vi "HEWH Data Cleanup at Index Location.vi"(10 "Test Data-Start to End IN":string[][](array[string]), 11 "Full Data DBL In":dbl[][](array[numeric])) -> (2 "Test Data-Start to End Out":string[][](array[string]), 3 "Full Data DBL Out":dbl[][](array[numeric]))   [LabVIEW 2020]
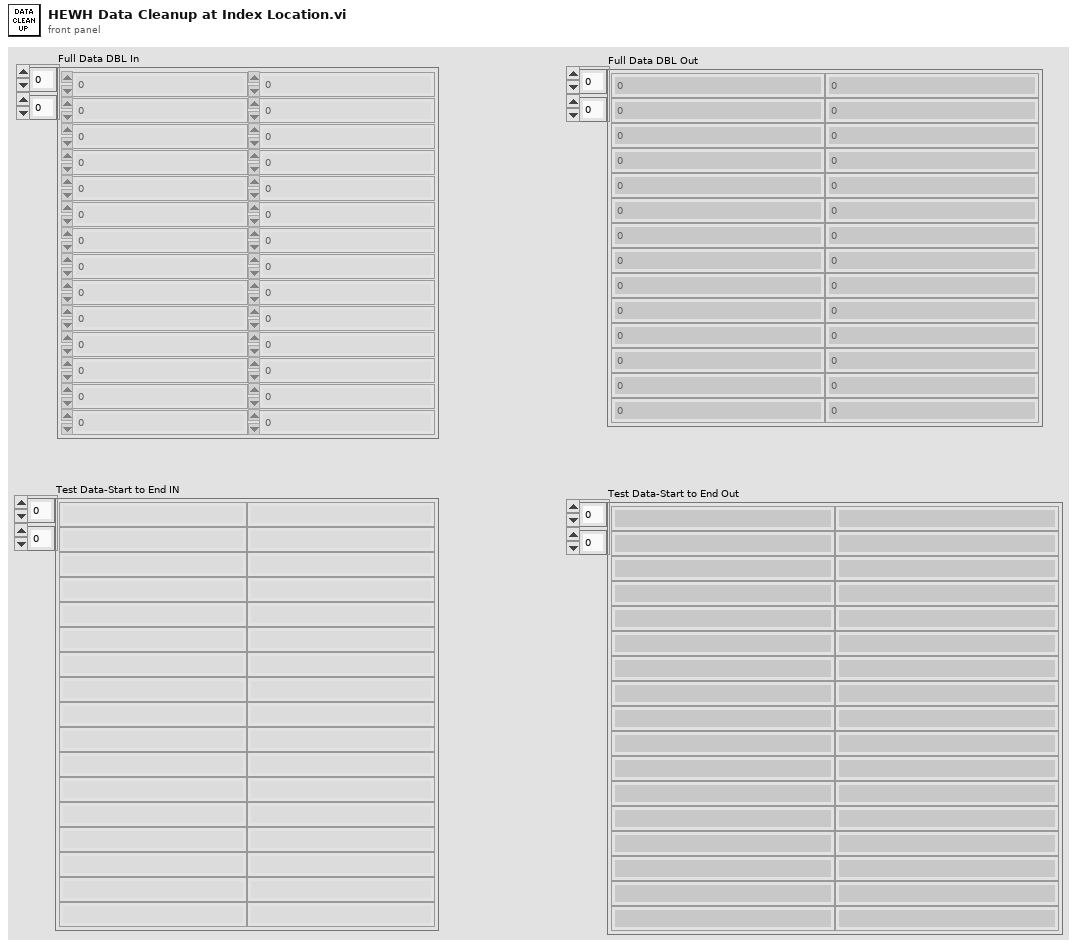
[diagram p1: front panel]
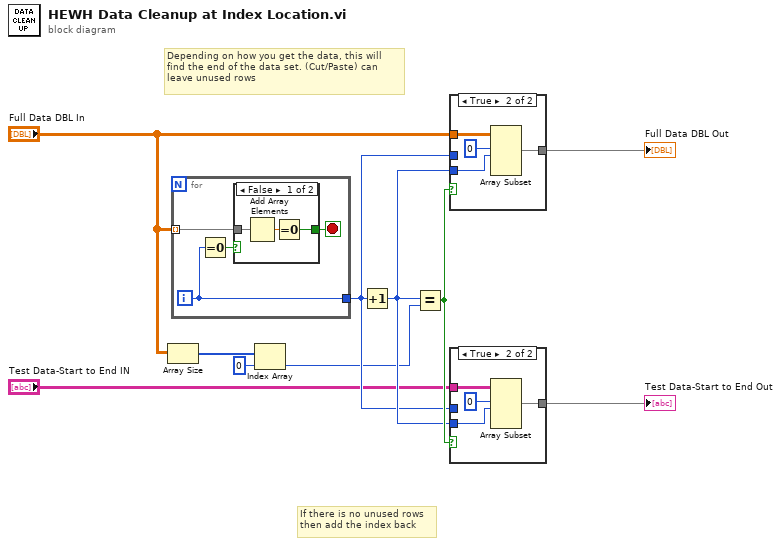
[diagram p0: block diagram]
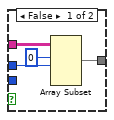
[diagram p2: hidden frame]
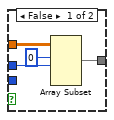
[diagram p3: hidden frame]
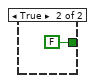
[diagram p4: hidden frame]
diagram:
  # "If there is no unused rows\nthen add the index back"
  # "Depending on how you get the data, this will\nfind the end of the data set. (Cut/Paste) can \nleave unused rows"
  n1 = Array Size(array="Full Data DBL In") -> (size(s)=w2:i32[])
  n2 = for {
    tunnel: "Full Data DBL In" -> [w11] mode=indexing
    tunnel: [w12] -> w6
    i -> [w12]
    stop <- w14 stop-if-true
    n3 = Equal To 0?(x=w12) -> (x = 0?=w13:bool)
    n4 = case shown="False" w13 {
      tunnel: w11 -> [w17 _]
      tunnel: [w16 FALSE] -> w14
      frame False {
        n5 = Add Array Elements(numeric array=w17) -> (sum=w15:dbl)
        n6 = Equal To 0?(x=w15) -> (x = 0?=w16:bool)
      }
      frame True {
      }
    }
  }
  n7 = Index Array(array=w2, index=0) -> (element=w4:i32)
  n8 = Increment(x=w6) -> (x+1=w7:i32)
  n9 = Equal?(x=w7, y=w4) -> (x = y?=w8:bool)
  n10 = case shown="True" w8 {
    tunnel: [w22 w24] -> w9
    tunnel: "Full Data DBL In" -> [w20 w26]
    tunnel: w6 -> [w19 _]
    tunnel: w7 -> [_ w23]
    frame False {
      n11 = Array Subset(array=w20, index (row)=0 ("index"), length (row)=w19) -> (w22:dbl[][])  [unwired: 2 in]
    }
    frame True {
      n12 = Array Subset(array=w26, index (row)=0 ("index"), length (row)=w23) -> (w24:dbl[][])  [unwired: 2 in]
    }
  }
  "Full Data DBL Out" <- w9
  n13 = case shown="True" w8 {
    tunnel: [w30 w32] -> w10
    tunnel: "Test Data-Start to End IN" -> [w28 w34]
    tunnel: w6 -> [w27 _]
    tunnel: w7 -> [_ w31]
    frame False {
      n14 = Array Subset(array=w28, index (row)=0 ("index"), length (row)=w27) -> (w30:string[][])  [unwired: 2 in]
    }
    frame True {
      n15 = Array Subset(array=w34, index (row)=0 ("index"), length (row)=w31) -> (w32:string[][])  [unwired: 2 in]
    }
  }
  "Test Data-Start to End Out" <- w10
